vi "set Packet Timeout.vi"(10 "packet_length":u16, 11 "port_num":i32) -> ()   [LabVIEW 2015, in "dxl_x86_c.lvlib"]
doc: "WINDECLSPEC void setPacketTimeout (int port_num, uint16_t packet_length);"
uses:
  dxl_x86_c.lvlib
  dxl_x86_c.dll
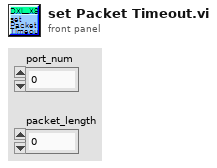
[diagram p1: front panel]
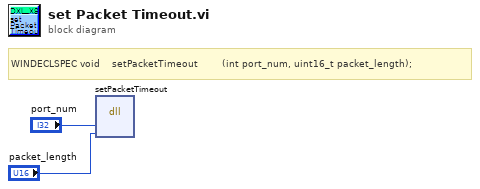
[diagram p0: block diagram]
diagram:
  # "WINDECLSPEC void    setPacketTimeout        (int port_num, uint16_t packet_length);"
  n1 = dll-call lib="C:/Users/Platform/Desktop/LabVIEW/dxl_x86_c.lvlib/dxl_x86_c.*" fn="setPacketTimeout"("port_num"="port_num", "packet_length"="packet_length") -> ()  [unwired: 6 in, 2 out]
